vi "table_set_subtable_item.vi"(4 "subkeys":string[](array[string]), 6 "close_item? (true)":bool=TRUE, 7 "subtables":string[](array[string]), 8 "error in (no error)":errorcluster, 9 "item (value)":refnum<class "Item.lvclass">, 10 "key":string, 11 "Table in":refnum<class "Table.lvclass">) -> (0 "error out":errorcluster, 3 "Table out":refnum<class "Table.lvclass">)   [LabVIEW 2020, in "toml.lvclass"]
uses:
  toml.lvclass
  Item/Item.lvclass
  Table/Table.lvclass
  toml.lvclass/toml.ctl
  InlineTable/InlineTable.lvclass
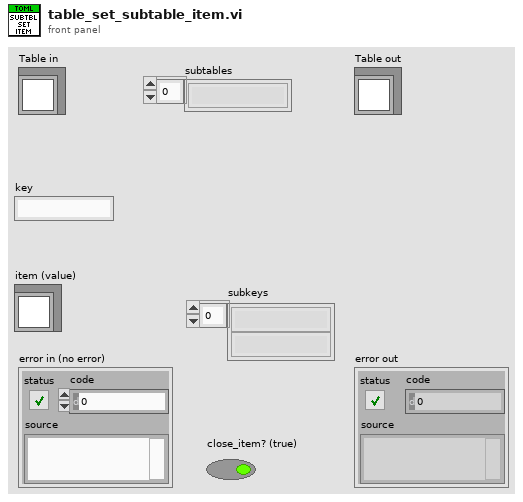
[diagram p1: front panel]
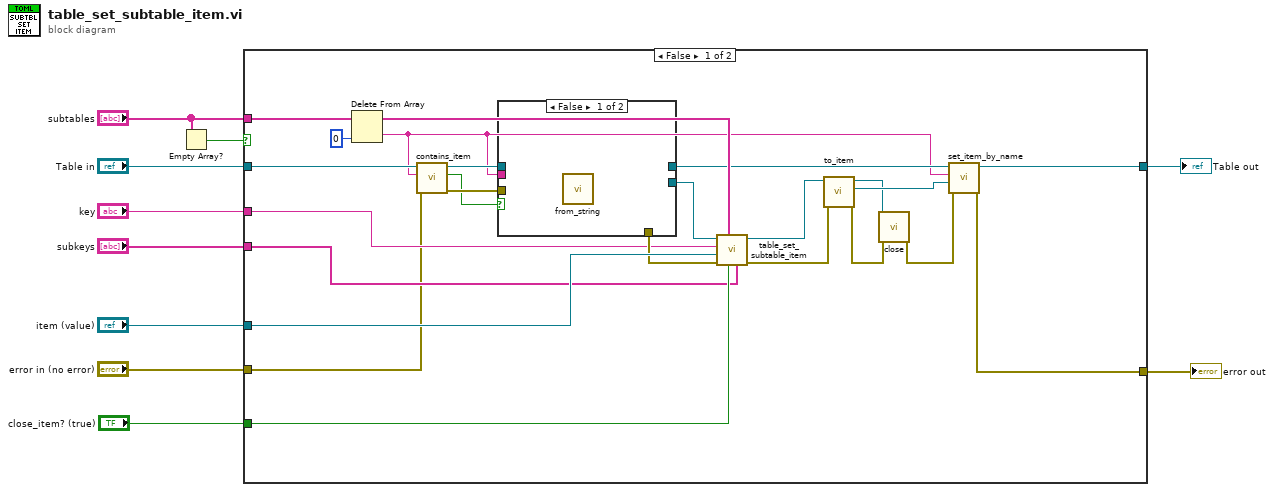
[diagram p0: block diagram]
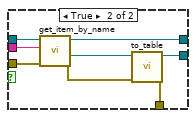
[diagram p2: hidden frame]
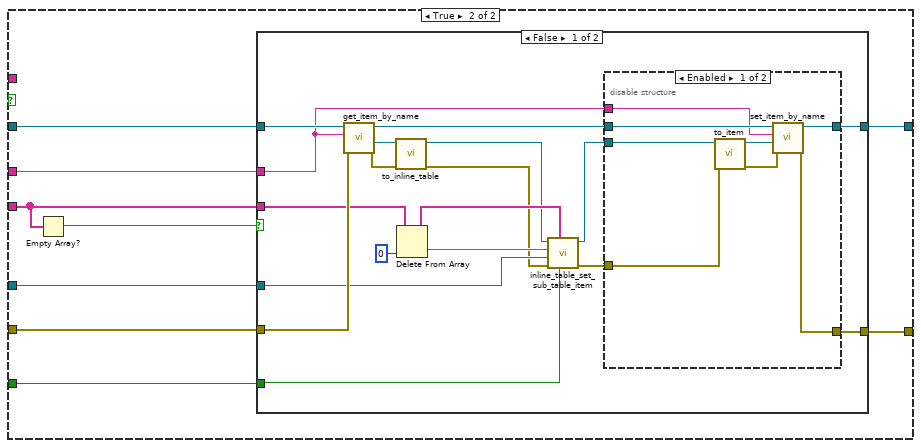
[diagram p3: hidden frame]
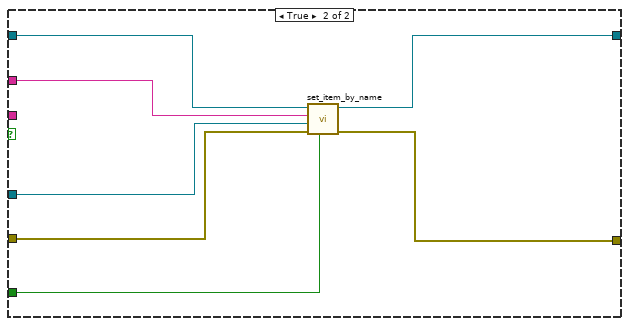
[diagram p5: hidden frame]
diagram:
  n1 = Empty Array?(array="subtables") -> (empty?=w4:bool)
  n2 = case shown="False" w4 {
    tunnel: [w27 w51] -> w10
    tunnel: "item (value)" -> [w29 w48]
    tunnel: "subkeys" -> [w17 w44]
    tunnel: [w20 w50] -> w7
    tunnel: "Table in" -> [w15 w49]
    tunnel: "error in (no error)" -> [w13 w47]
    tunnel: "subtables" -> [w34 _]
    tunnel: "close_item? (true)" -> [w19 w46]
    tunnel: "key" -> [w18 w43]
    frame False {
      n3 = Delete From Array(array=w34, index=0) -> (deleted portion=w12:string, array with subset deleted=w32:string[])  [unwired: 1 in]
      n4 = call "contains_item.vi"("error in (no error)"=w13, "item_name"=w12, "Table in"=w15) -> ("error out"=w14:errorcluster, "contains_item"=w11:bool, "Table out"=w16:refnum<class "Table.lvclass">)  [unwired: 6 in]
      n5 = case shown="False" w11 {
        tunnel: [_ w41] -> w31
        tunnel: [_ w40] -> w30
        tunnel: [_ w39] -> w28
        tunnel: w16 -> [_ w37]
        tunnel: w14 -> [_ w36]
        tunnel: w12 -> [_ w35]
        frame False {
          n6 = call "from_string.vi"() -> ()  [unwired: 10 in, 2 out]
        }
        frame True {
          n7 = call "get_item_by_name.vi"("error in (no error)"=w36, "item_name"=w35, "Table in"=w37) -> ("error out"=w38:errorcluster, "Item"=w42:refnum<class "Item.lvclass">, "Table out"=w41:refnum<class "Table.lvclass">)  [unwired: 6 in]
          n8 = call "to_table.vi"("error in (no error)"=w38, "Item in"=w42) -> ("error out"=w39:errorcluster, "Table"=w40:refnum<class "Table.lvclass">)  [unwired: 8 in]
        }
      }
      n9 = call "table_set_subtable_item.vi"("subkeys"=w17, "close_item? (true)"=w19, "subtables"=w32, "error in (no error)"=w28, "item (value)"=w29, "key"=w18, "Table in"=w30) -> ("error out"=w24:errorcluster, "Table out"=w25:refnum<class "Table.lvclass">)  [unwired: 3 in]
      n10 = call "to_item.vi"("error in (no error)"=w24, "Table in"=w25) -> ("error out"=w22:errorcluster, "Item out"=w26:refnum<class "Item.lvclass">, "Table out"=w23:refnum<class "Table.lvclass">)  [unwired: 7 in]
      n11 = call "close.vi"("error in (no error)"=w22, "Table in"=w23) -> ("error out"=w21:errorcluster)  [unwired: 9 in]
      n12 = call "set_item_by_name.vi"("error in (no error)"=w21, "Item"=w26, "item_name"=w12, "Table in"=w31) -> ("error out"=w27:errorcluster, "Table out"=w20:refnum<class "Table.lvclass">)  [unwired: 6 in]
    }
    frame True {
      n13 = Empty Array?(array=w44) -> (empty?=w45:bool)
      n14 = case shown="False" w45 {
        tunnel: [w57 w86] -> w51
        tunnel: [w58 w85] -> w50
        tunnel: w49 -> [w68 w84]
        tunnel: w48 -> [w59 w83]
        tunnel: w47 -> [w67 w82]
        tunnel: w46 -> [w56 w81]
        tunnel: w44 -> [w61 _]
        tunnel: w43 -> [w64 w80]
        frame False {
          n15 = call "get_item_by_name.vi"("error in (no error)"=w67, "item_name"=w64, "Table in"=w68) -> ("error out"=w54:errorcluster, "Item"=w55:refnum<class "Item.lvclass">, "Table out"=w69:refnum<class "Table.lvclass">)  [unwired: 6 in]
          n16 = call "to_inline_table.vi"("error in (no error)"=w54, "Item in"=w55) -> ("error out"=w53:errorcluster, "InlineTable"=w52:refnum<class "InlineTable.lvclass">)  [unwired: 8 in]
          n17 = Delete From Array(array=w61, index=0) -> (deleted portion=w60:string, array with subset deleted=w62:string[])  [unwired: 1 in]
          n18 = call "inline_table_set_sub_table_item.vi"("close_item? (true)"=w56, "subtables"=w62, "error in (no error)"=w53, "item (value)"=w59, "key"=w60, "InlineTable in"=w52) -> ("error out"=w66:errorcluster, "InlineTable out"=w65:refnum<class "InlineTable.lvclass">)  [unwired: 4 in]
          n19 = disable-structure shown="Enabled" {
            disable-tunnel: w69 -> [w77 w79]
            disable-tunnel: [w76 w79] -> w58
            disable-tunnel: [w75 w78] -> w57
            disable-tunnel: w66 -> [w74 w78]
            disable-tunnel: w65 -> [w73 _]
            disable-tunnel: w64 -> [w72 _]
            frame Enabled {
              n20 = call "to_item.vi"("error in (no error)"=w74, "Table in"=w73) -> ("error out"=w71:errorcluster, "Item out"=w70:refnum<class "Item.lvclass">)  [unwired: 8 in]
              n21 = call "set_item_by_name.vi"("error in (no error)"=w71, "Item"=w70, "item_name"=w72, "Table in"=w77) -> ("error out"=w75:errorcluster, "Table out"=w76:refnum<class "Table.lvclass">)  [unwired: 6 in]
            }
            frame Disabled {
            }
          }
        }
        frame True {
          n22 = call "set_item_by_name.vi"("close_item? (true)"=w81, "error in (no error)"=w82, "Item"=w83, "item_name"=w80, "Table in"=w84) -> ("error out"=w86:errorcluster, "Table out"=w85:refnum<class "Table.lvclass">)  [unwired: 5 in]
        }
      }
    }
  }
  "error out" <- w10
  "Table out" <- w7
